vi "Find Closest Direction.vi"(11 "Angle":dbl format="%#_13g") -> (3 "Closest Angle":dbl)   [LabVIEW 2017]
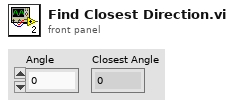
[diagram p1: front panel]
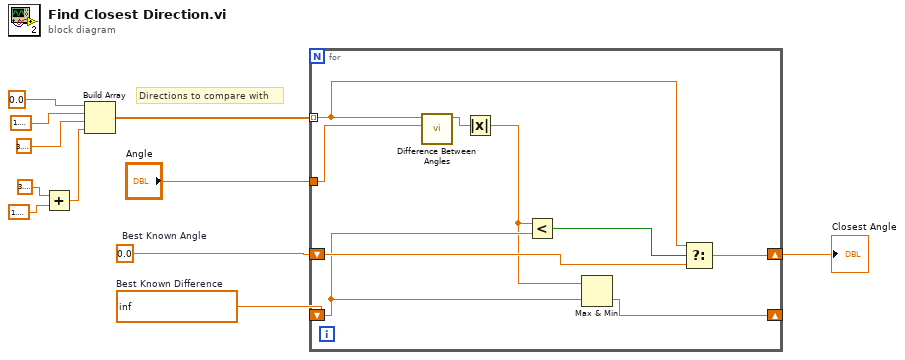
[diagram p0: block diagram]
diagram:
  w3 = 0.0  # Best Known Angle
  w2 = inf  # Best Known Difference
  # "Directions to compare with"
  n1 = Add(x=3.141592653589793, y=1.5707963267948966) -> (x+y=w6:dbl)
  n2 = Build Array(0.0 ("element"), 1.5707963267948966, 3.141592653589793, w6) -> (w5:dbl[])
  n3 = for {
    tunnel: w5 -> [w14] mode=indexing
    tunnel: "Angle" -> [w19]
    shift-right: [w17] -> w1
    shift-left: w3 -> [w18]
    shift-right: [w15] -> _
    shift-left: w2 -> [w16]
    n4 = call "Difference Between Angles.vi"("Angle 2"=w19, "Angle 1"=w14) -> ("Difference"=w13:dbl)  [unwired: 9 in]
    n5 = Absolute Value(x=w13) -> (abs(x)=w12:dbl)
    n6 = Less?(x=w12, y=w16) -> (x < y?=w20:bool)
    n7 = Max & Min(x=w12, y=w16) -> (min(x,y)=w15:dbl)  [unwired: 1 out]
    n8 = Select(t=w14, s=w20, f=w18) -> (s? t:f=w17:dbl)
  }
  "Closest Angle" <- w1
